vi "Excel Easy Table (num).vi"(0 "report in":refnum<class "NI_report.lvclass">, 1 "iteration":i32, 2 "font":T1={"font name"="", "font size"=10.0, "bold"=0, "italic"=0, "underline"=0, "strike through"=0, "font color"=16777216} {"font size" format="%0.2f"; "strike through" items=["Unchanged", "Yes", "No"]; "underline" items=["Unchanged", "Yes", "No"]; "italic" items=["Unchanged", "Yes", "No"]; "bold" items=["Unchanged", "Yes", "No"]}, 3 "font settings source":u16(ring) items=["VI Inputs", "Font Dialog Box"], 5 "auto format (none)":i32(ring)=-4142 items=["xlRangeAutoFormat3DEffects1"=13, "xlRangeAutoFormat3DEffects2"=14, "xlRangeAutoFormatAccounting1"=4, "xlRangeAutoFormatAccounting2"=5, "xlRangeAutoFormatAccounting3"=6, "xlRangeAutoFormatAccounting4"=17, "xlRangeAutoFormatClassic1"=1, "xlRangeAutoFormatClassic2"=2, "xlRangeAutoFormatClassic3"=3, "xlRangeAutoFormatColor1"=7, "xlRangeAutoFormatColor2"=8, "xlRangeAutoFormatColor3"=9, "xlRangeAutoFormatList1"=10, "xlRangeAutoFormatList2"=11, "xlRangeAutoFormatList3"=12, "xlRangeAutoFormatLocalFormat1"=15, "xlRangeAutoFormatLocalFormat2"=16, "xlRangeAutoFormatLocalFormat3"=19, "xlRangeAutoFormatLocalFormat4"=20, "xlRangeAutoFormatReport1"=21, "xlRangeAutoFormatReport2"=22, "xlRangeAutoFormatReport3"=23, "xlRangeAutoFormatReport4"=24, "xlRangeAutoFormatReport5"=25, "xlRangeAutoFormatReport6"=26, "xlRangeAutoFormatReport7"=27, "xlRangeAutoFormatReport8"=28, "xlRangeAutoFormatReport9"=29, "xlRangeAutoFormatReport10"=30, "xlRangeAutoFormatClassicPivotTable"=31, "xlRangeAutoFormatTable1"=32, "xlRangeAutoFormatTable2"=33, "xlRangeAutoFormatTable3"=34, "xlRangeAutoFormatTable4"=35, "xlRangeAutoFormatTable5"=36, "xlRangeAutoFormatTable6"=37, "xlRangeAutoFormatTable7"=38, "xlRangeAutoFormatTable8"=39, "xlRangeAutoFormatTable9"=40, "xlRangeAutoFormatTable10"=41, "xlRangeAutoFormatPTNone"=42, "xlRangeAutoFormatNone"=-4142, "xlRangeAutoFormatSimple"=-4154], 7 "start (0, 0)":cluster{"row":i32, "column":i32}, 9 "text data":dbl[][](array[numeric]) format="%0.2f", 11 "error in (no error)":errorcluster, 12 "name (\"\")":string, 13 "row headers":string[](array[string]), 14 "column headers":string[](array[string])) -> (4 "report out":refnum<class "NI_report.lvclass">, 6 "font out":T1={"font name"="", "font size"=10.0, "bold"=0, "italic"=0, "underline"=0, "strike through"=0, "font color"=16777216} {"font size" format="%0.2f"; "strike through" items=["Unchanged", "Yes", "No"]; "underline" items=["Unchanged", "Yes", "No"]; "italic" items=["Unchanged", "Yes", "No"]; "bold" items=["Unchanged", "Yes", "No"]}, 8 "next cell bottom-left":cluster{"row":i32, "column":i32}, 10 "next cell top-right":cluster{"row":i32, "column":i32}, 15 "error out":errorcluster)   [LabVIEW 2017, in "NI_ReportGenerationToolkit.lvlib"]
doc: "Inserts and formats a table into a Microsoft Excel report. The data type you wire to the <B>text data</B> input determines the polymorphic instance to use."
uses:
  <vilib>/addons/_office/NI_ReportGenerationToolkit.lvlib
  <vilib>/Utility/NIReport.llb/NI_report.lvclass
  <vilib>/addons/_office/_exclsub.llb/font.ctl
  <vilib>/Utility/NIReport.llb/Append Numeric Table to Report (wrap).vi
  <vilib>/Utility/NIReport.llb/Excel/NI_Excel.lvclass
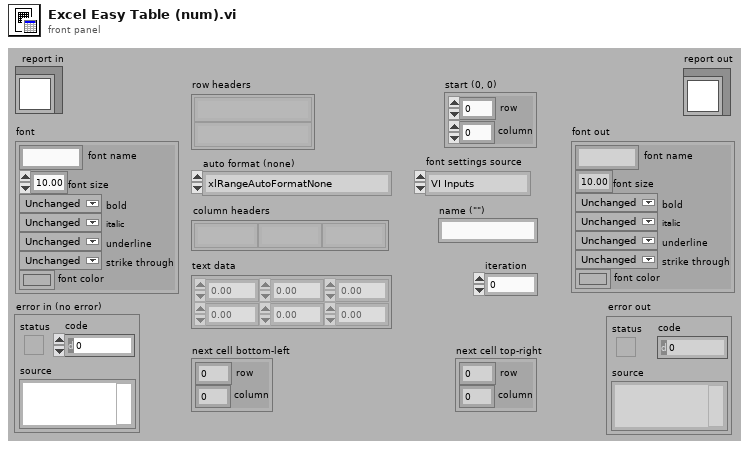
[diagram p1: front panel]
types:
  T1 = typedef "NI_ReportGenerationToolkit.lvlib/font.ctl" = cluster{"font name":string, "font size":dbl, "bold":u16, "italic":u16, "underline":u16, "strike through":u16, "font color":u32}
  T2 = cluster{"Charset (-1)":i16, "Weight (-1)":i16, "Name":string, "Size":string}
  T3 = cluster{"position (Excel)":cluster{"row":i32, "column":i32}, "name (Excel)":string, "bookmark (Word)":string}
  T4 = cluster{i32, i32, i32, i32, "charset":i16, "weight":i16, "name":string, "size":string, "text color":u32}
  T5 = cluster{"italic":u16, "strike through":u16, "underline":u16, "bold":u16}
  T6 = typedef "NI_ReportGenerationCore.lvlib/font.ctl" = cluster{"font name":string, "font size":dbl, "bold":u16, "italic":u16, "underline":u16, "strike through":u16, "font color":u32}
  T7 = cluster{"start (wd) - row (xl) ":i32, "end (wd) - col (xl) ":i32}
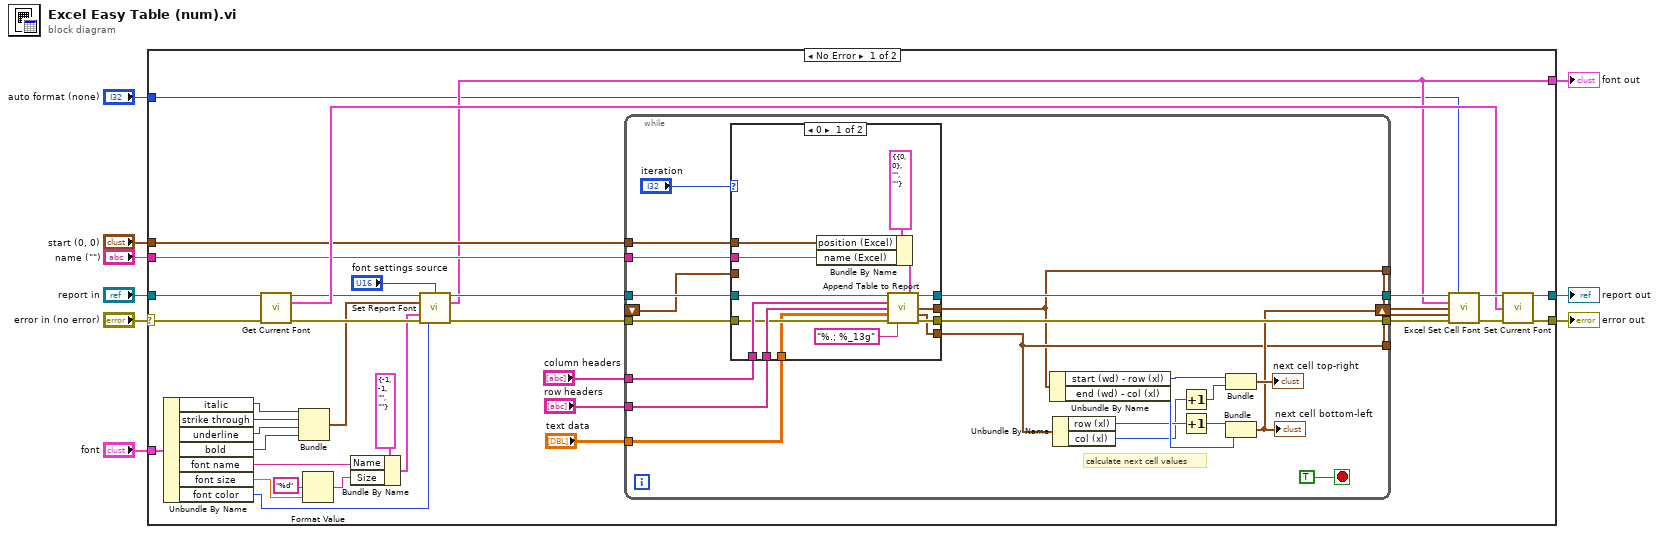
[diagram p0: block diagram]
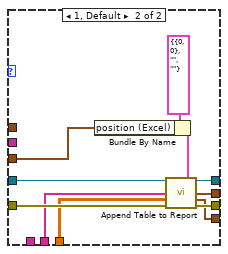
[diagram p2: hidden frame]
diagram:
  n1 = case shown="No Error" "error in (no error)" {
    selector: "error in (no error)" -> [w13 w93]
    tunnel: "report in" -> [w43 w94]
    tunnel: [w40 w93] -> w8
    tunnel: [w39 w94] -> w7
    tunnel: "start (0, 0)" -> [w37 _]
    tunnel: "name (\"\")" -> [w36 _]
    tunnel: "font" -> [w18 _]
    tunnel: [w11 _] -> w2
    tunnel: "auto format (none)" -> [w10 _]
    frame No Error {
      n2 = Unbundle By Name(w18) -> ("italic"=w25:u16, "strike through"=w24:u16, "underline"=w23:u16, "bold"=w22:u16, "font name"=w26:string, "font size"=w20:dbl, "font color"=w17:u32)
      n3 = call <vilib>:"Get Current Font.vi"("report in"=w43, "error in (no error)"=w13) -> ("report.lvclass"=w29:refnum<class "NI_report.lvclass">, "font"=w38:T4, "error out"=w31:errorcluster)  [unwired: 11 out]
      n4 = Bundle("italic"=w25, "strike through"=w24, "underline"=w23, "bold"=w22) -> (w15:T5)  [unwired: 1 out]
      n5 = Format Value(format string="%d", value (0)=w20) -> (output string=w19:string)  [unwired: 1 out]
      n6 = Bundle By Name(cluster=T2 {"Charset (-1)"=-1, "Weight (-1)"=-1, "Name"="", "Size"=""} ("font settings"), "Name"=w26, "Size"=w19) -> (w16:T2)
      n7 = call-dynamic "Set Report Font.vi"("report in"=w29, "text color (unchanged)"=w17, "font settings source (VI Inputs)"="font settings source", "text options"=w15, "font settings"=w16, "error in (no error)"=w31) -> ("report out"=w28:refnum<class "NI_report.lvclass">, "font out"=w11:T6, "error out"=w30:errorcluster)  [unwired: 7 in]
      n8 = while {
        tunnel: [w67] -> w45
        tunnel: [w66] -> w44
        tunnel: w28 -> [w65]
        tunnel: w30 -> [w64]
        tunnel: w37 -> [w63]
        tunnel: w36 -> [w62]
        shift-right: [w51] -> _
        shift-left: _ -> [w60]
        tunnel: [w46] -> w12
        tunnel: [w50] -> w35
        tunnel: "row headers" -> [w49]
        tunnel: "column headers" -> [w48]
        tunnel: "text data" -> [w47]
        stop <- TRUE stop-if-true
        # "calculate next cell values"
        n9 = case shown="0" "iteration" {
          tunnel: w48 -> [w81 _]
          tunnel: w49 -> [w80 w86]
          tunnel: [w79 w90] -> w67
          tunnel: [w78 w89] -> w66
          tunnel: [w75 w84] -> w50
          tunnel: w65 -> [w74 w87]
          tunnel: w64 -> [w73 w88]
          tunnel: w63 -> [w72 _]
          tunnel: w62 -> [w71 _]
          tunnel: [w70 w85] -> w46
          tunnel: w60 -> [_ w83]
          tunnel: w47 -> [w69 w82]
          frame 0 {
            n10 = Bundle By Name(cluster=T3 {"position (Excel)"={"row"=0, "column"=0}, "name (Excel)"="", "bookmark (Word)"=""} ("MS Office parameters"), "position (Excel)"=w72, "name (Excel)"=w71) -> (w76:T3)
            n11 = call-poly <vilib>:"Append Table to Report.vi"("report in"=w74, "MS Office parameters"=w76, "column headers"=w81, "row headers"=w80, "numerical data"=w69, "error in (no error)"=w73, "format string (%.3f)"="%.; %_13g") -> ("report out"=w79:refnum<class "NI_report.lvclass">, "range (wd) - start (xl)"=w70:T7, "end (xl)"=w75:cluster{"row (xl) ":i32, "col (xl) ":i32}, "error out"=w78:errorcluster)  [unwired: 3 in, 2 out]
          }
          frame 1, Default {
            n12 = Bundle By Name(cluster=T3 {"position (Excel)"={"row"=0, "column"=0}, "name (Excel)"="", "bookmark (Word)"=""} ("MS Office parameters"), "position (Excel)"=w83) -> (w91:T3)
            n13 = call-poly <vilib>:"Append Table to Report.vi"("report in"=w87, "MS Office parameters"=w91, "row headers"=w86, "numerical data"=w82, "error in (no error)"=w88) -> ("report out"=w90:refnum<class "NI_report.lvclass">, "range (wd) - start (xl)"=w85:T7, "end (xl)"=w84:cluster{"row (xl) ":i32, "col (xl) ":i32}, "error out"=w89:errorcluster)  [unwired: 5 in, 2 out]
          }
        }
        n14 = Unbundle By Name(w46) -> ("start (wd) - row (xl)"=w52:i32, "end (wd) - col (xl)"=w58:i32)
        n15 = Unbundle By Name(w50) -> ("row (xl)"=w56:i32, "col (xl)"=w53:i32)
        n16 = Increment(x=w53) -> (x+1=w54:i32)
        n17 = Increment(x=w56) -> (x+1=w57:i32)
        n18 = Bundle("start (wd) - row (xl)"=w52, w54) -> (→"next cell top-right":cluster{"start (wd) - row (xl) ":i32, i32})  [unwired: 1 out]
        n19 = Bundle(w57, "end (wd) - col (xl)"=w58) -> (w51:cluster{i32, "end (wd) - col (xl) ":i32})  [unwired: 1 out]
        "next cell bottom-left" <- w51
      }
      n20 = call <vilib>:"Excel Set Cell Font.vi"("report in"=w45, "auto format"=w10, "font"=w11, "start (-1, -1)"=w12, "end (-1, -1)"=w35, "error in (no error)"=w44) -> ("report out"=w41:refnum<class "NI_report.lvclass">, "error out"=w42:errorcluster)  [unwired: 8 out]
      n21 = call <vilib>:"Set Current Font.vi"("report in"=w41, "font"=w38, "error in (no error)"=w42) -> ("report out"=w39:refnum<class "NI_report.lvclass">, "error out"=w40:errorcluster)  [unwired: 11 out]
    }
    frame Error {
    }
  }
  "error out" <- w8
  "report out" <- w7
  "font out" <- w2
